vi "Read Roles.vi"(8 "error in (no error)":errorcluster, 11 "PreparePassInGame1 in":refnum<class "PreparePassInGame1.lvclass">) -> (0 "error out":errorcluster, 2 "Roles":T1, 3 "PreparePassInGame1 out":refnum<class "PreparePassInGame1.lvclass">)   [LabVIEW 2021, in "PreparePassInGame1.lvclass"]
uses:
  PreparePassInGame1.lvclass
  ShootRole_class/ShootRole.lvclass
  PreparePassReceiverRole_class/PreparePassReceiverRole.lvclass
  PreparePassInGame1.lvclass/PreparePassInGame1.ctl
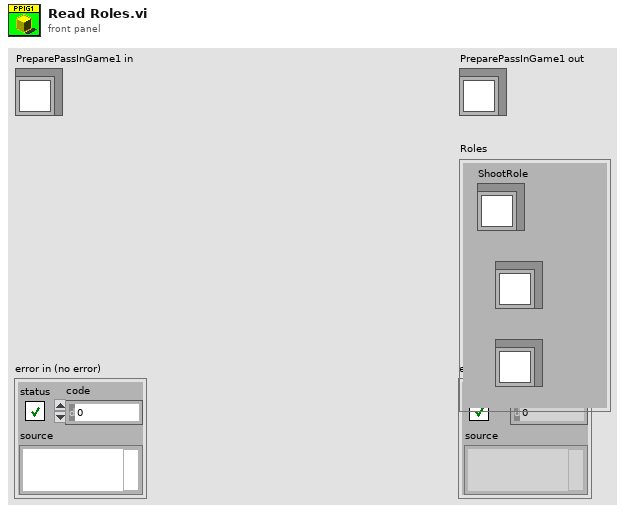
[diagram p1: front panel]
types:
  T1 = cluster{"ShootRole":refnum<class "ShootRole.lvclass">, "PreparePassReceiverRole1":refnum<class "PreparePassReceiverRole.lvclass">, "PreparePassReceiverRole2":refnum<class "PreparePassReceiverRole.lvclass">}
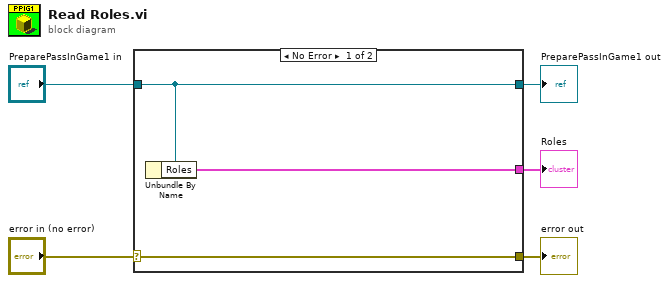
[diagram p0: block diagram]
diagram:
  n1 = case shown="No Error" "error in (no error)" {
    selector: "error in (no error)" -> [w8 w9]
    tunnel: [w8 w9] -> w4
    tunnel: [w7 w10] -> w2
    tunnel: "PreparePassInGame1 in" -> [w7 w10]
    tunnel: [w6 _] -> w1
    frame No Error {
      n2 = Unbundle By Name(w7) -> ("Roles"=w6:T1)
    }
    frame Error {
    }
  }
  "error out" <- w4
  "PreparePassInGame1 out" <- w2
  "Roles" <- w1
